vi "test2.vi"() -> ()   [LabVIEW 2014]
uses:
  picohrdl.dll
panel:
  out "Sensor3":i32[](graph)
  in  "1 5":bool=TRUE
  in  "1 4":bool=TRUE
  in  "1 3":bool=TRUE
  in  "1 2":bool=TRUE
  in  "1":bool=TRUE
  in  "conversionTime":i16(ring) items=["60 ms", "100 ms", "180 ms", "340 ms", "660 ms"]
  in  "Mains Frequency":i16(ring) items=["50 Hz", "60 Hz"]
  out "Waveform Graph 3":dynamicdata(graph)
  in  "sampleInterval_ms":i32=1000
  in  "stop":bool
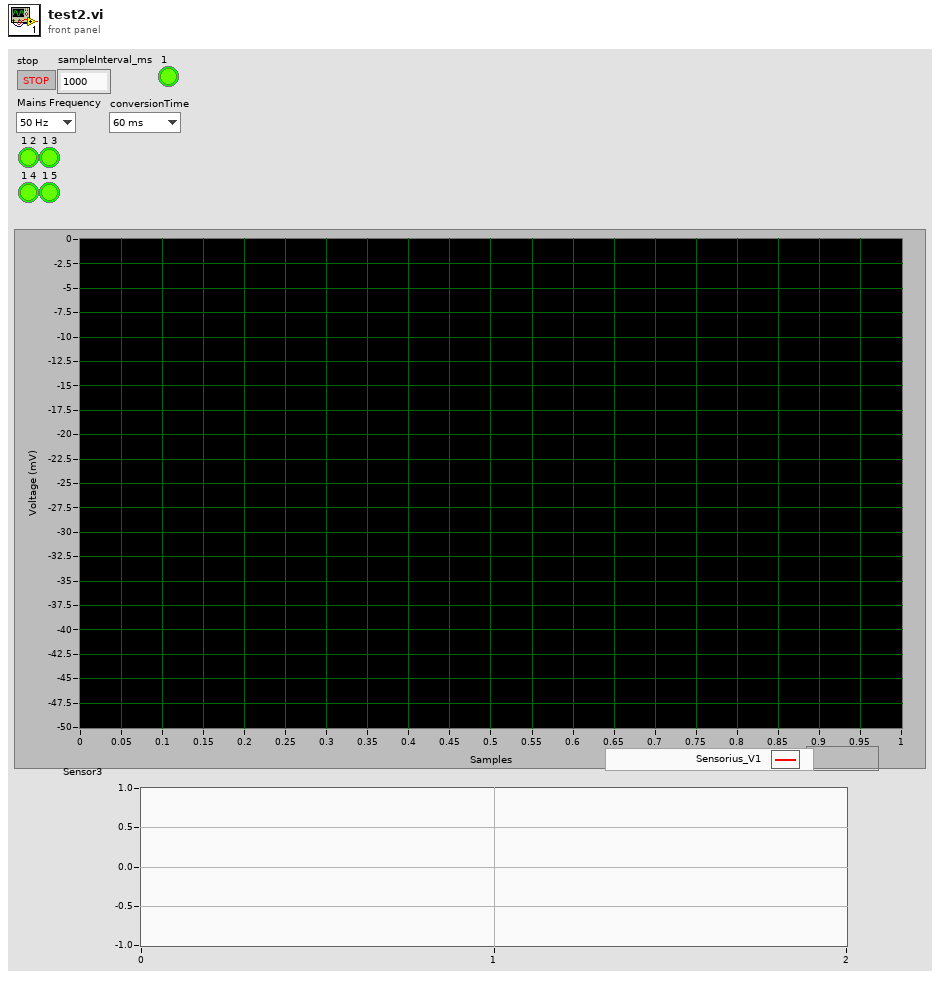
[diagram p1: front panel]
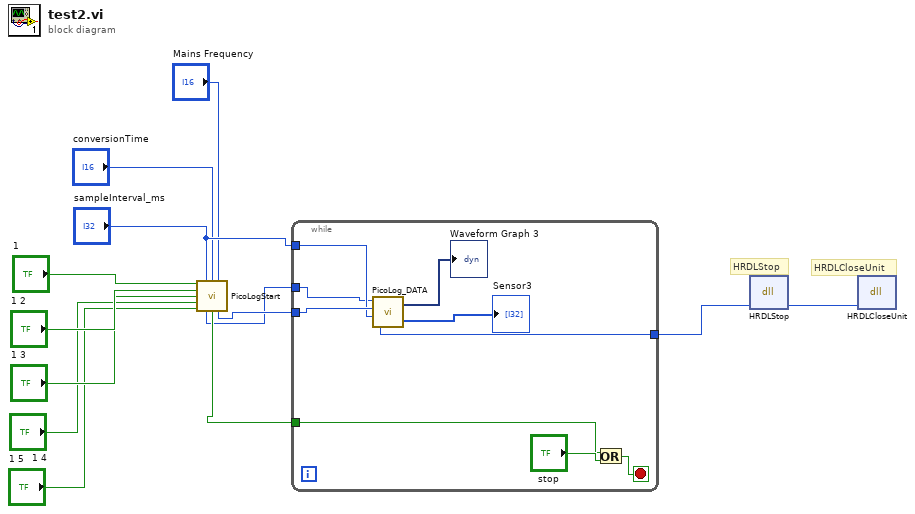
[diagram p0: block diagram]
diagram:
  # "HRDLStop"
  # "HRDLCloseUnit"
  n1 = call "PicoLogStart.vi"(0:"1", "sampleInterval_ms"="sampleInterval_ms", "conversionTime"="conversionTime", "Mains Frequency"="Mains Frequency", 5:"1 2", 7:"1 3", "4"="1 4", "5"="1 5") -> ("noOfChannels"=w1:i16, "STOP"=w4:bool, "handle"=w13:i16)  [unwired: 5 in]
  n2 = while {
    tunnel: w13 -> [w22]
    tunnel: "sampleInterval_ms" -> [w21]
    tunnel: w4 -> [w17]
    tunnel: [w16] -> w2
    tunnel: w1 -> [w15]
    stop <- w19 stop-if-true
    n3 = call "PicoLog_DATA.vi"("sampleInterval_ms"=w21, "handle"=w22, "noOfChannels"=w15) -> ("Sensor3"=→"Sensor3":i32[], "Waveform Graph 3"=→"Waveform Graph 3":dynamicdata, "handle"=w16:i16)
    n4 = Or(x=w17, y="stop") -> (x .or. y?=w19:bool)
  }
  n5 = dll-call lib="picohrdl.dll" fn="HRDLStop"("handle"=w2) -> ("handle"=w3:i16)  [unwired: 4 in, 2 out]
  n6 = dll-call lib="PicoHRDL.dll" fn="HRDLCloseUnit"("handle"=w3) -> ()  [unwired: 5 in, 2 out]
